vi "Put (NT Enum (Index)).vi"(6 "timestamp in":timestamp, 7 "PV name":string, 8 "error in (no error)":errorcluster, 9 "timeout":dbl[unit]=1.0, 10 "index in":u16, 11 "Client in":refnum<class "Client.lvclass">) -> (0 "error out":errorcluster, 1 "timed out?":bool, 2 "index out":u16, 3 "Client out":refnum<class "Client.lvclass">, 4 "timestamp out":timestamp)   [LabVIEW 2020, in "PV Access.lvlib" / "PVA Client.lvlib" / "Client.lvclass"]
uses:
  Client.lvclass
  PV Data/PV Data/Write Field (I32).vi
  PV Data/PV Data/PV Data.lvclass
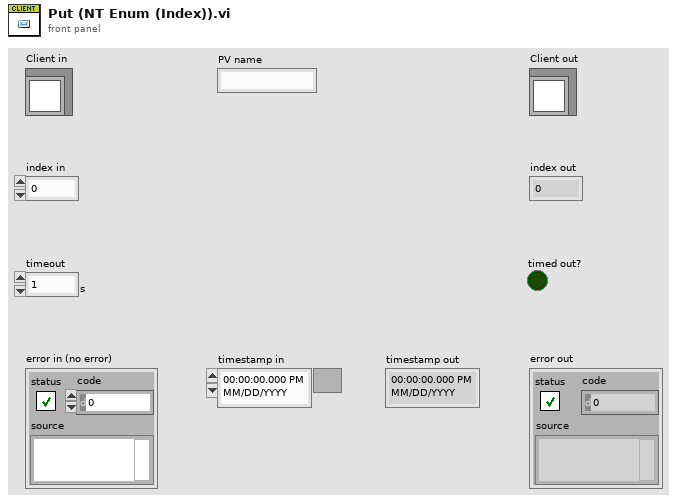
[diagram p1: front panel]
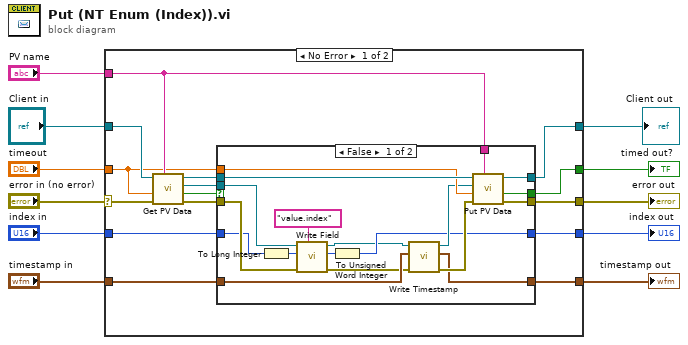
[diagram p0: block diagram]
diagram:
  n1 = case shown="No Error" "error in (no error)" {
    selector: "error in (no error)" -> [w24 w54]
    tunnel: [w23 w54] -> w4
    tunnel: [w22 w53] -> w5
    tunnel: "Client in" -> [w25 w53]
    tunnel: "PV name" -> [w21 _]
    tunnel: "timeout" -> [w19 _]
    tunnel: "index in" -> [w12 w51]
    tunnel: [w17 w51] -> w1
    tunnel: [w15 _] -> w6
    tunnel: "timestamp in" -> [w14 w52]
    tunnel: [w13 w52] -> w3
    frame No Error {
      n2 = call "Get PV Data.vi"("PV name"=w21, "error in"=w24, "timeout"=w19, "Client in"=w25) -> ("error out"=w18:errorcluster, "timed out?"=w16:bool, "PV Data out"=w20:refnum<class "PV Data.lvclass">, "Client out"=w26:refnum<class "Client.lvclass">)  [unwired: 4 in]
      n3 = case shown="False" w16 {
        selector: w16 -> [_ w49]
        tunnel: w26 -> [w45 w48]
        tunnel: [w44 w50] -> w23
        tunnel: [w43 w48] -> w22
        tunnel: w21 -> [w42 _]
        tunnel: w20 -> [w41 _]
        tunnel: w19 -> [w40 _]
        tunnel: w18 -> [w39 w50]
        tunnel: [w29 w46] -> w17
        tunnel: [w38 w49] -> w15
        tunnel: w14 -> [w36 w47]
        tunnel: [w34 w47] -> w13
        tunnel: w12 -> [w31 w46]
        frame False {
          n4 = To Long Integer(number=w31) -> (32bit integer=w32:i32)
          n5 = call-poly "Write Field.vi"("field name"="value.index", "error in"=w39, "value"=w32, "PV Data in"=w41) -> ("error out"=w28:errorcluster, "value out"=w30:i32, "PV Data out"=w27:refnum<class "PV Data.lvclass">)  [unwired: 5 in]
          n6 = To Unsigned Word Integer(number=w30) -> (unsigned 16bit integer=w29:u16)
          n7 = call "Write Timestamp.vi"("error in"=w28, "timestamp in"=w36, "PV Data in"=w27) -> ("error out"=w35:errorcluster, "timestamp out"=w34:timestamp, "PV Data out"=w37:refnum<class "PV Data.lvclass">)  [unwired: 5 in, 1 out]
          n8 = call "Put PV Data.vi"("PV name"=w42, "error in"=w35, "timeout"=w40, "PV Data in"=w37, "Client in"=w45) -> ("error out"=w44:errorcluster, "timed out?"=w38:bool, "Client out"=w43:refnum<class "Client.lvclass">)  [unwired: 4 in]
        }
        frame True {
        }
      }
    }
    frame Error {
    }
  }
  "error out" <- w4
  "Client out" <- w5
  "timed out?" <- w6
  "timestamp out" <- w3
  "index out" <- w1
